vi "Display Lab Panel V5.vi"() -> ()   [LabVIEW 2013]
uses:
  Global display 1.vi
  Global display 2.vi
  Global display 3.vi
panel:
  in  "Tab Control 2":T1(tab)
  out "SIG LAB05-2":T2 {"PF" format="%.2f"; "AMPS" format="%.1f"}
  out "SIG LAB05-1":T2 {"PF" format="%.2f"; "AMPS" format="%.1f"}
  out "SIG LAB04-2":T2 {"PF" format="%.2f"; "AMPS" format="%.1f"}
  out "SIG LAB04-1":T2 {"PF" format="%.2f"; "AMPS" format="%.1f"}
  out "SIG LAB03-2":T2 {"PF" format="%.2f"; "AMPS" format="%.1f"}
  out "SIG LAB03-1":T2 {"PF" format="%.2f"; "AMPS" format="%.1f"}
  out "SIG LAB02-2":T2 {"PF" format="%.2f"; "AMPS" format="%.1f"}
  in  "RUN LAB01-1":bool
  in  "O/I  LAB05-1":bool
  in  "O/I  LAB05-2":bool
  in  "O/I  LAB04-1":bool
  in  "O/I  LAB04-2":bool
  in  "O/I  LAB02-1":bool
  in  "O/I  LAB02-2":bool
  in  "O/I  LAB01-2":bool
  in  "O/I  LAB01-1":bool
  in  "O/I  LAB03-1":bool
  in  "RUN LAB05-2":bool
  in  "RUN LAB05-1":bool
  in  "RUN LAB04-2":bool
  in  "RUN LAB04-1":bool
  in  "RUN LAB03-2":bool
  in  "RUN LAB03-1":bool
  in  "RUN LAB02-2":bool
  in  "RUN LAB02-1":bool
  in  "RUN LAB01-2":bool
  in  "SELECT LAB05-2":T3(radio)
  in  "SELECT LAB05-1":T3(radio)
  in  "SELECT LAB04-2":T3(radio)
  in  "SELECT LAB04-1":T3(radio)
  in  "SELECT LAB03-2":T3(radio)
  in  "SELECT LAB03-1":T3(radio)
  in  "SELECT LAB02-2":T3(radio)
  in  "SELECT LAB02-1":T3(radio)
  in  "SELECT LAB01-2":T3(radio)
  in  "SELECT LAB01-1":T3(radio)
  in  "O/I  LAB03-2":bool
  out "SIG LAB01-1":T2 {"PF" format="%.2f"; "AMPS" format="%.1f"}
  out "SIG LAB01-2":T2 {"PF" format="%.2f"; "AMPS" format="%.1f"}
  out "SIG LAB02-1":T2 {"PF" format="%.2f"; "AMPS" format="%.1f"}
  out "DISP LAB05-2":T4 {"MINS" format="%.2g"}
  out "DISP LAB05-1":T4 {"MINS" format="%.2g"}
  out "DISP LAB04-2":T4 {"MINS" format="%.2g"}
  out "DISP LAB04-1":T4 {"MINS" format="%.2g"}
  out "DISP LAB03-2":T4 {"MINS" format="%.2g"}
  out "DISP LAB03-1":T4 {"MINS" format="%.2g"}
  in  "SET LAB05-2":T5={"NAME"="", "DESCRIPTION"="", "CYCLES"=5.0, "T-RISE mins"=0.0, "T-RISE deg C"=0.0} {"CYCLES" min=5.0 step=1.0}
  in  "SET LAB05-1":T5={"NAME"="", "DESCRIPTION"="", "CYCLES"=5.0, "T-RISE mins"=0.0, "T-RISE deg C"=0.0} {"CYCLES" min=5.0 step=1.0}
  in  "SET LAB04-2":T5={"NAME"="", "DESCRIPTION"="", "CYCLES"=5.0, "T-RISE mins"=0.0, "T-RISE deg C"=0.0} {"CYCLES" min=5.0 step=1.0}
  in  "SET LAB04-1":T5={"NAME"="", "DESCRIPTION"="", "CYCLES"=5.0, "T-RISE mins"=0.0, "T-RISE deg C"=0.0} {"CYCLES" min=5.0 step=1.0}
  in  "SET LAB03-2":T5={"NAME"="", "DESCRIPTION"="", "CYCLES"=5.0, "T-RISE mins"=0.0, "T-RISE deg C"=0.0} {"CYCLES" min=5.0 step=1.0}
  in  "SET LAB03-1":T5={"NAME"="", "DESCRIPTION"="", "CYCLES"=5.0, "T-RISE mins"=0.0, "T-RISE deg C"=0.0} {"CYCLES" min=5.0 step=1.0}
  out "DISP LAB02-2":T4 {"MINS" format="%.2g"}
  out "DISP LAB02-1":T4 {"MINS" format="%.2g"}
  in  "SET LAB02-2":T5={"NAME"="", "DESCRIPTION"="", "CYCLES"=5.0, "T-RISE mins"=0.0, "T-RISE deg C"=0.0} {"CYCLES" min=5.0 step=1.0}
  in  "SET LAB02-1":T5={"NAME"="", "DESCRIPTION"="", "CYCLES"=5.0, "T-RISE mins"=0.0, "T-RISE deg C"=0.0} {"CYCLES" min=5.0 step=1.0}
  out "RESULT LAB05-2":bool
  out "RESULT LAB05-1":bool
  out "RESULT LAB04-2":bool
  out "RESULT LAB04-1":bool
  out "RESULT LAB03-2":bool
  out "RESULT LAB03-1":bool
  out "RESULT LAB02-2":bool
  out "RESULT LAB02-1":bool
  out "RESULT LAB01-2":bool
  out "RESULT LAB01-1":bool
  in  "SET LAB01-1":T5={"NAME"="", "DESCRIPTION"="", "CYCLES"=5.0, "T-RISE mins"=0.0, "T-RISE deg C"=0.0} {"CYCLES" min=5.0 step=1.0}
  in  "SET LAB01-2":T5={"NAME"="", "DESCRIPTION"="", "CYCLES"=5.0, "T-RISE mins"=0.0, "T-RISE deg C"=0.0} {"CYCLES" min=5.0 step=1.0}
  out "DISP LAB01-1":T4 {"MINS" format="%.2g"}
  out "DISP LAB01-2":T4 {"MINS" format="%.2f"}
  in  "Save Log Files\nTo Disk For\nViewing":bool
  out "LOG LAB05-2":string
  out "LOG LAB04-2":string
  out "LOG LAB03-2":string
  out "LOG LAB02-2":string
  out "LOG LAB01-2":string
  out "LOG LAB05-1":string
  out "LOG LAB04-1":string
  out "LOG LAB03-1":string
  out "LOG LAB02-1":string
  out "LOG LAB01-1":string
  out "LAB01 TEMP":dynamicdata(graph)
  out "LAB01 VOLTS":dynamicdata(graph)
  out "LAB01 AMPS":dynamicdata(graph)
  out "LAB02 TEMP":dynamicdata(graph)
  out "LAB02 VOLTS":dynamicdata(graph)
  out "LAB02 AMPS":dynamicdata(graph)
  out "LAB03 TEMP":dynamicdata(graph)
  out "LAB03 VOLTS":dynamicdata(graph)
  out "LAB03 AMPS":dynamicdata(graph)
  out "LAB04 TEMP":dynamicdata(graph)
  out "LAB04 VOLTS":dynamicdata(graph)
  out "LAB04 AMPS":dynamicdata(graph)
  out "LAB05 TEMP":dynamicdata(graph)
  out "LAB05 VOLTS":dynamicdata(graph)
  out "LAB05 AMPS":dynamicdata(graph)
  in  "Stop Button":bool
  out "log file dir":string
  out "log5-2":dbl
  out "log4-2":dbl
  out "log3-2":dbl
  out "log2-2":dbl
  out "log1-2":dbl
  out "log5-1":dbl
  out "log4-1":dbl
  out "log3-1":dbl
  out "log2-1":dbl
  out "log1-1":dbl
  out "graph update":bool
  out "LF5-2":bool
  out "LF5-1":bool
  out "LF3-2":bool
  out "LF3-1":bool
  out "LF4-2":bool
  out "LF4-1":bool
  out "LF2-2":bool
  out "LF2-1":bool
  out "LF1-2":bool
  out "LF1-1":bool
  out "error out":errorcluster
  # "LAB01"
  # "LAB02"
  # "LAB05"
  # "LAB03"
  # "LAB04"
  # "LAB01"
  # "LAB02"
  # "LAB03"
  # "LAB04"
  # "LAB05"
  # "PANEL ID / DATE / TIME / DESCRIPTION / CYCLES / TEST TIME / STATUS"
  # "PANEL ID / DATE / TIME / DESCRIPTION / CYCLES / TEST TIME / STATUS"
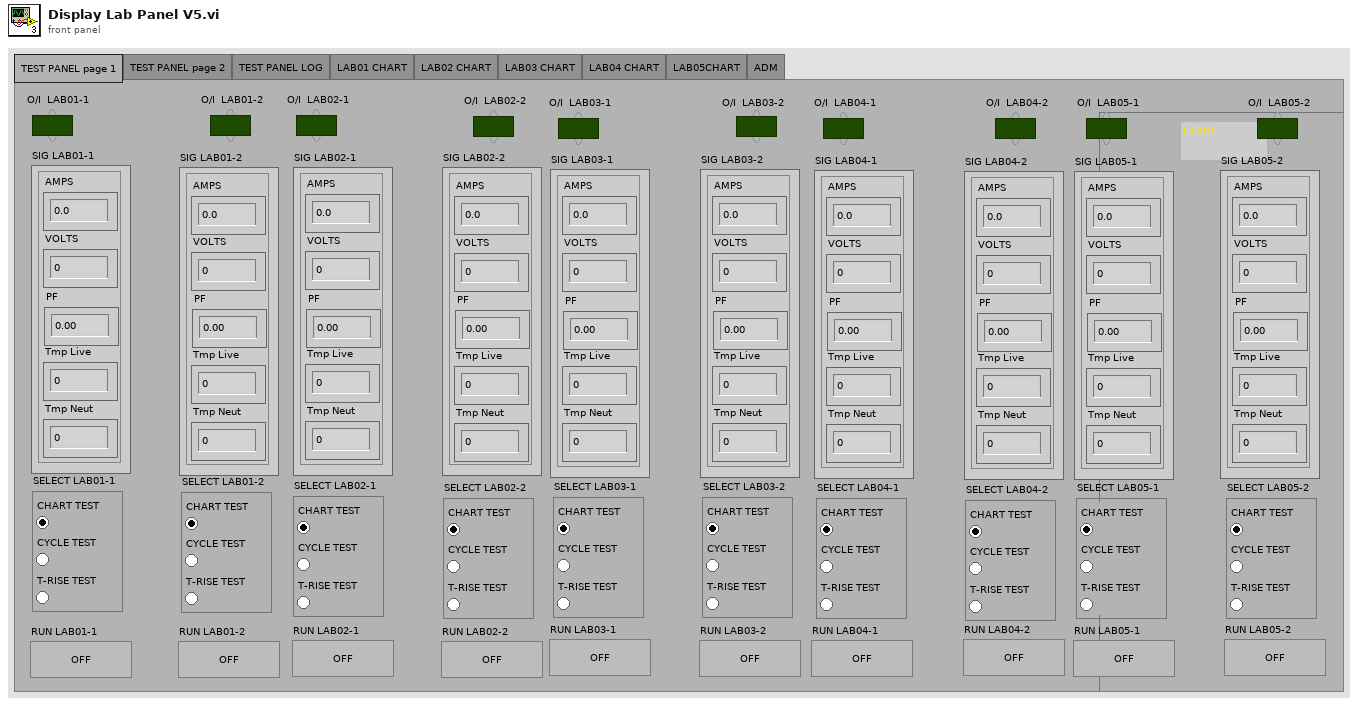
[diagram p1: front panel]
types:
  T1 = enum32{"TEST PANEL page 1", "TEST PANEL page 2", "TEST PANEL LOG", "LAB01 CHART", "LAB02 CHART", "LAB03 CHART", "LAB04 CHART", "LAB05CHART", "ADM"}
  T2 = cluster{"AMPS":dbl, "VOLTS":dbl, "PF":dbl, "Tmp Live":dbl, "Tmp Neut":dbl}
  T3 = enum32{"CHART TEST", "CYCLE TEST", "T-RISE TEST"}
  T4 = cluster{"CYCLE":dbl, "MINS":dbl, "STATUS":string}
  T5 = cluster{"NAME":string, "DESCRIPTION":string, "CYCLES":dbl, "T-RISE mins":dbl, "T-RISE deg C":dbl}
  T6 = enum8{"Enabled", "Disabled", "Disabled and Grayed Out"}
  T7 = cluster{string, "date string":string, "time string":string, "DESCRIPTION":string, string, string, "STATUS":string}
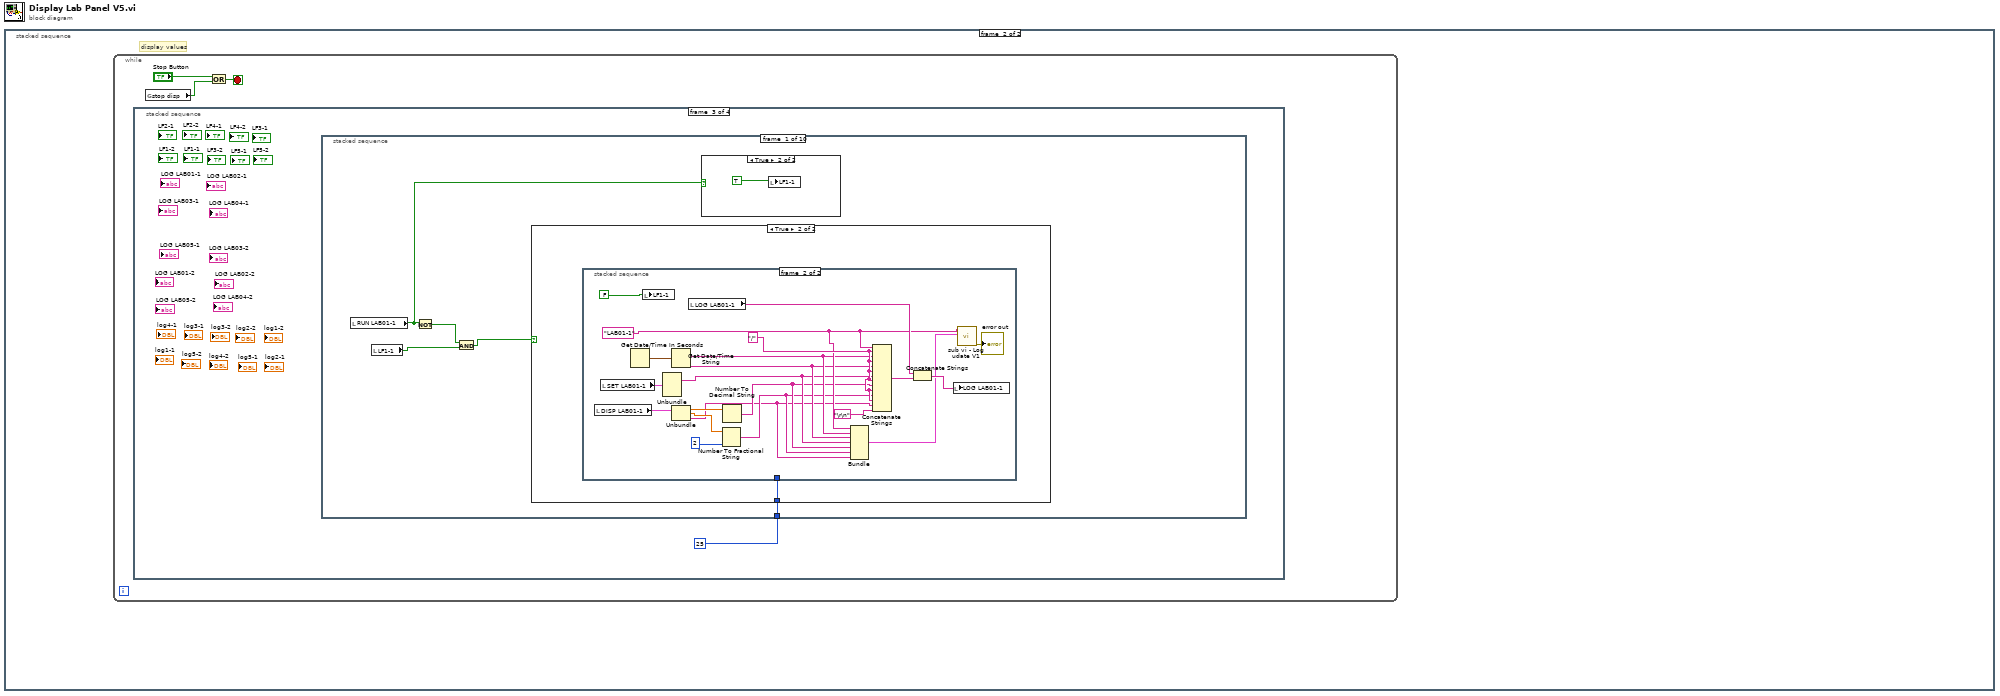
[diagram p0: block diagram]
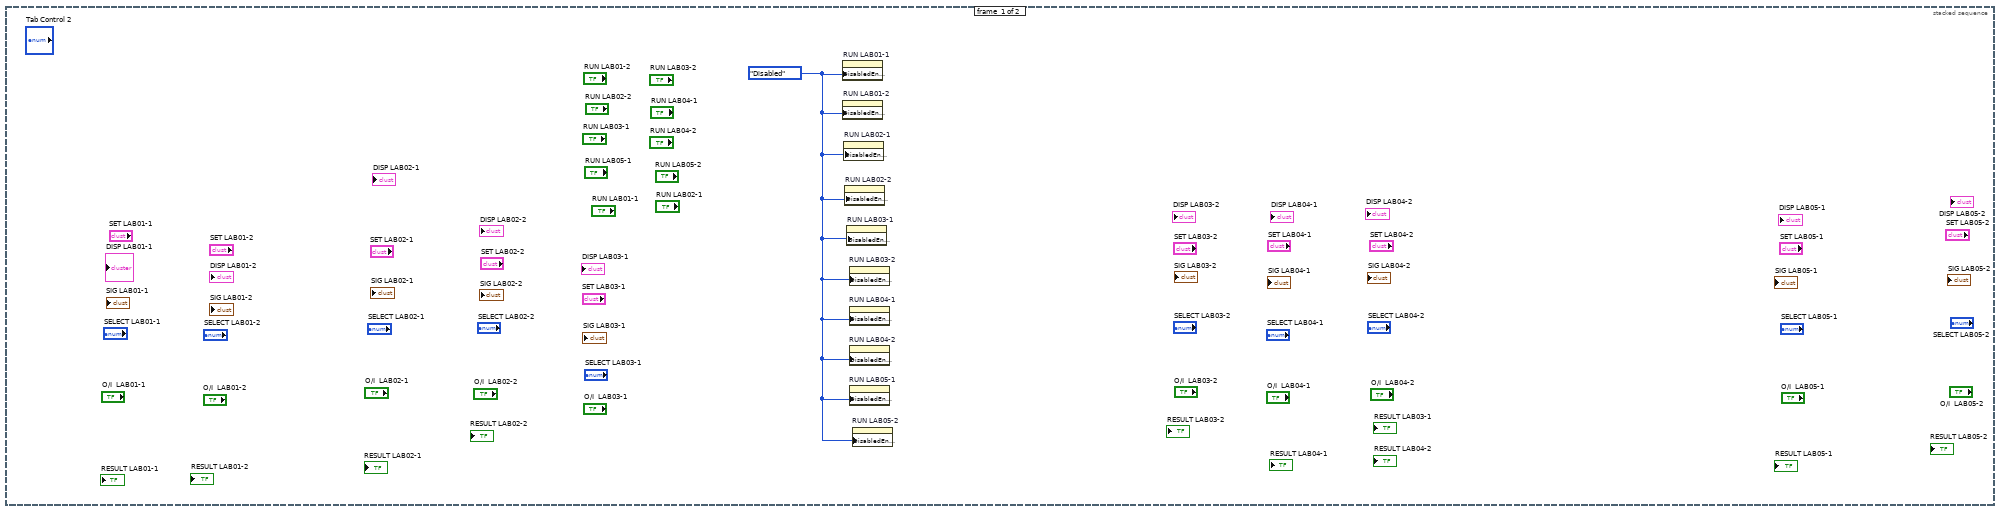
[diagram p2: hidden frame]
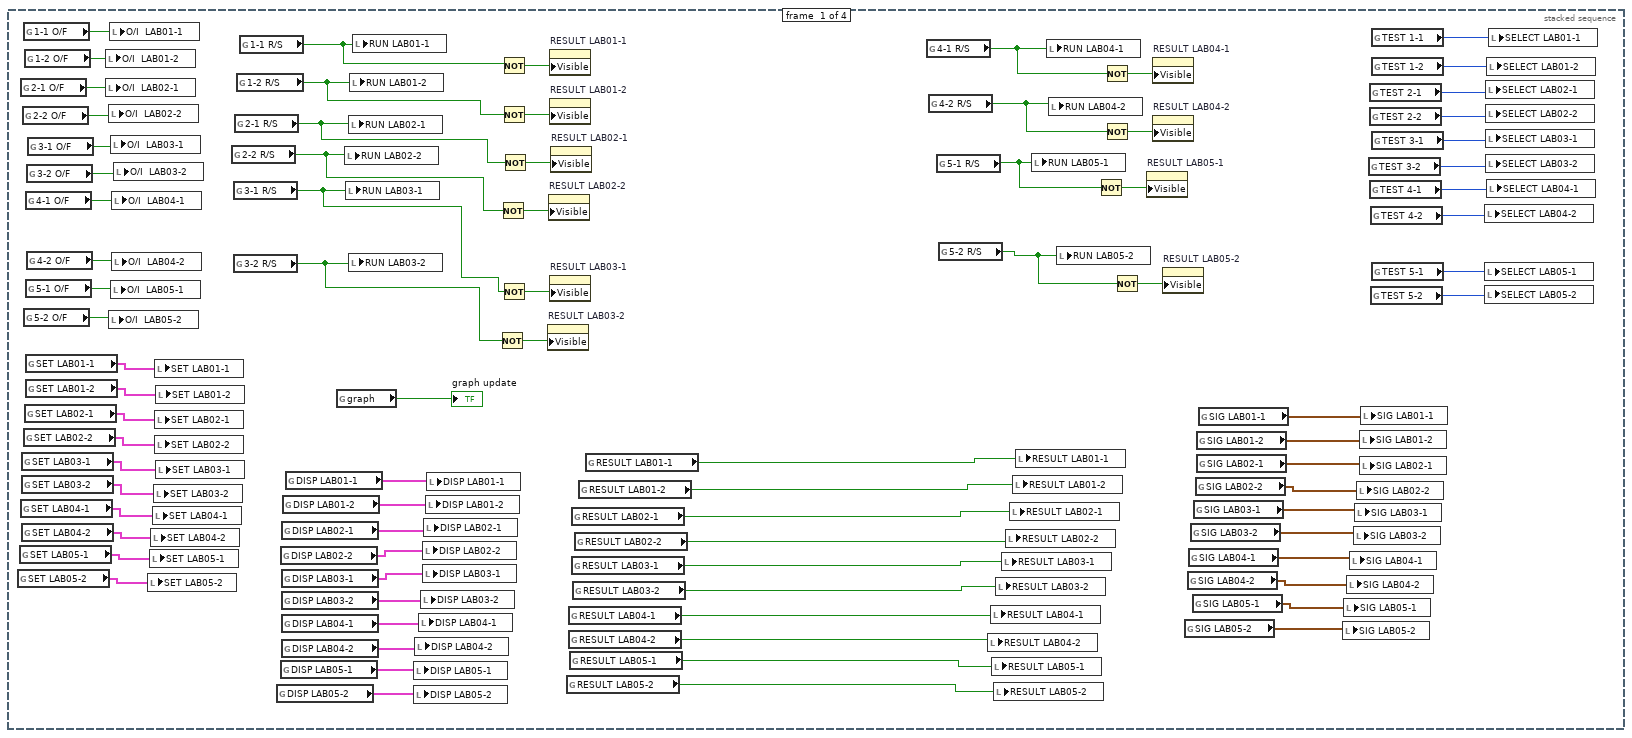
[diagram p3: hidden frame]
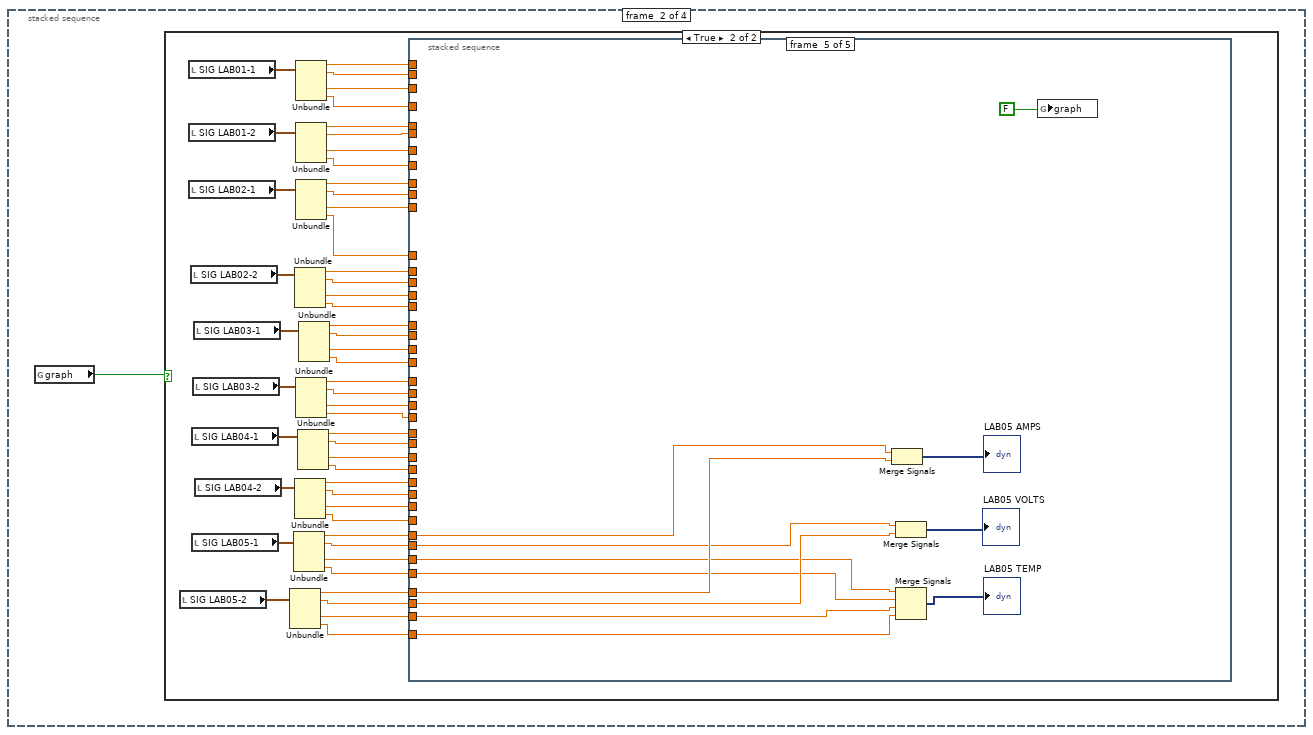
[diagram p4: hidden frame]
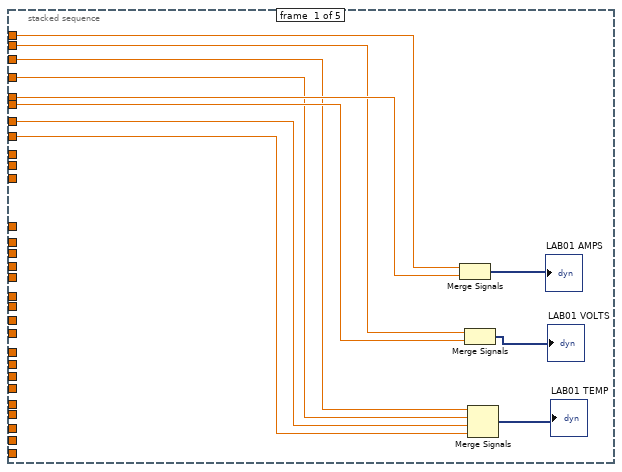
[diagram p6: hidden frame]
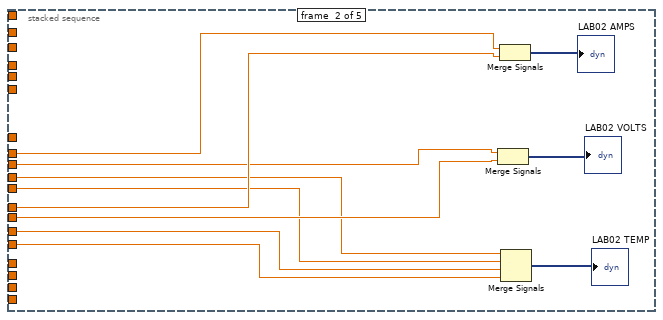
[diagram p7: hidden frame]
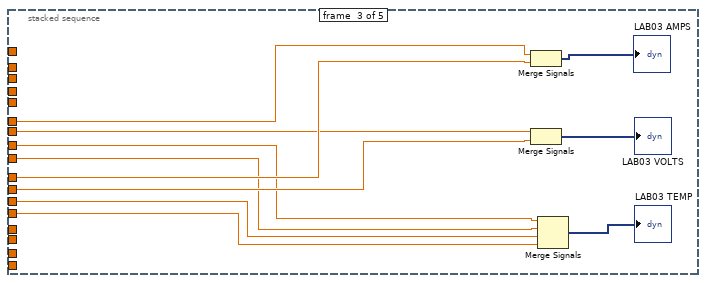
[diagram p8: hidden frame]
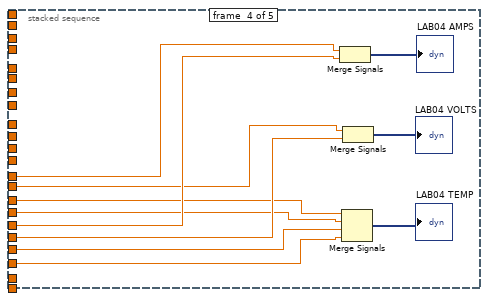
[diagram p9: hidden frame]
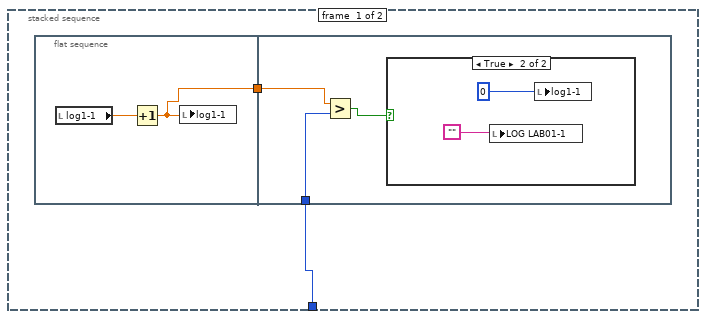
[diagram p11: hidden frame]
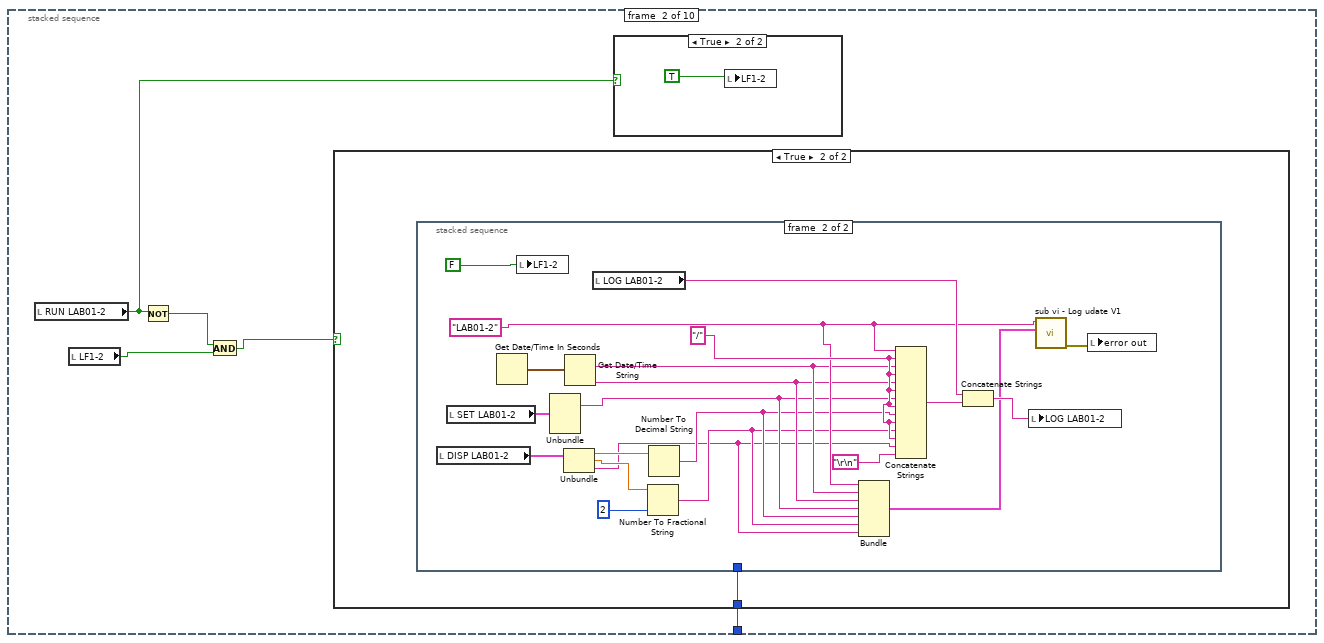
[diagram p14: hidden frame]
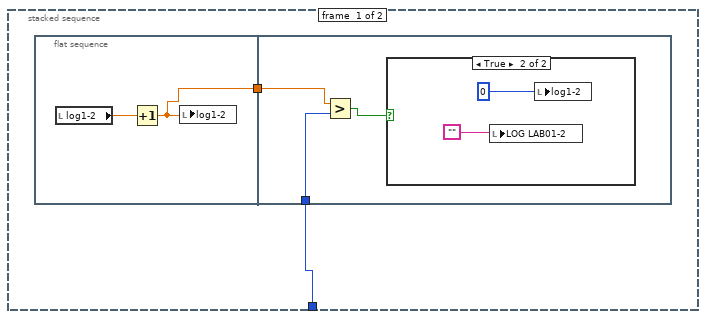
[diagram p16: hidden frame]
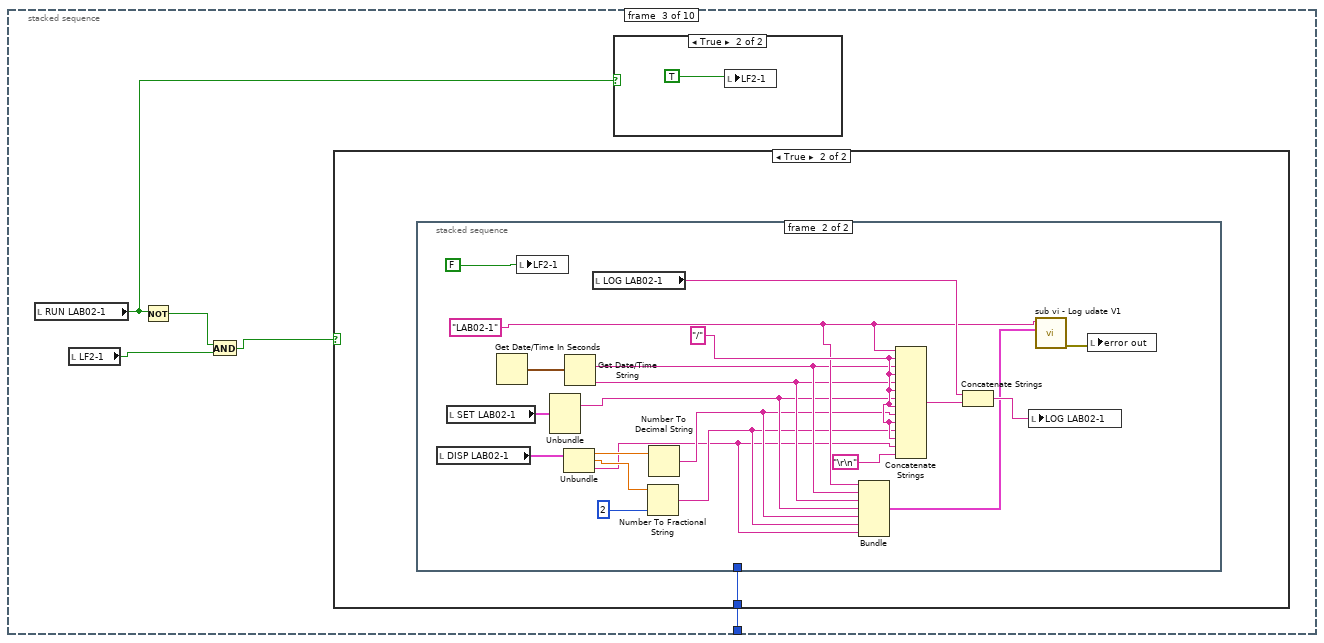
[diagram p19: hidden frame]
diagram:
  n1 = stacked-sequence {
    frame #0 {
      w1 = T6."Disabled" ("Disabled")
      n2 = property on="RUN LAB01-1" class="Bool (strict)"("DisabledEnum"=w1) -> ()  [unwired: 2 in, 2 out]
      n3 = property on="RUN LAB01-2" class="Bool (strict)"("DisabledEnum"=w1) -> ()  [unwired: 2 in, 2 out]
      n4 = property on="RUN LAB02-1" class="Bool (strict)"("DisabledEnum"=w1) -> ()  [unwired: 2 in, 2 out]
      n5 = property on="RUN LAB02-2" class="Bool (strict)"("DisabledEnum"=w1) -> ()  [unwired: 2 in, 2 out]
      n6 = property on="RUN LAB03-1" class="Bool (strict)"("DisabledEnum"=w1) -> ()  [unwired: 2 in, 2 out]
      n7 = property on="RUN LAB03-2" class="Bool (strict)"("DisabledEnum"=w1) -> ()  [unwired: 2 in, 2 out]
      n8 = property on="RUN LAB04-1" class="Bool (strict)"("DisabledEnum"=w1) -> ()  [unwired: 2 in, 2 out]
      n9 = property on="RUN LAB04-2" class="Bool (strict)"("DisabledEnum"=w1) -> ()  [unwired: 2 in, 2 out]
      n10 = property on="RUN LAB05-1" class="Bool (strict)"("DisabledEnum"=w1) -> ()  [unwired: 2 in, 2 out]
      n11 = property on="RUN LAB05-2" class="Bool (strict)"("DisabledEnum"=w1) -> ()  [unwired: 2 in, 2 out]
    }
    frame #1 {
      # "display values"
      n12 = while {
        stop <- w4 stop-if-true
        n13 = stacked-sequence {
          frame #0 {
            n14 = global read "Global display 2.vi" "SET LAB05-2"() -> (w46:T5)
            n15 = global read "Global display 2.vi" "SET LAB05-1"() -> (w47:T5)
            n16 = global read "Global display 1.vi" "2-1 O/F"() -> (w83:bool)
            n17 = global read "Global display 2.vi" "SET LAB04-1"() -> (w49:T5)
            n18 = global read "Global display 2.vi" "SET LAB03-1"() -> (w51:T5)
            n19 = global read "Global display 2.vi" "SET LAB03-2"() -> (w50:T5)
            n20 = global read "Global display 2.vi" "SET LAB04-2"() -> (w48:T5)
            n21 = global read "Global display 1.vi" "2-2 O/F"() -> (w82:bool)
            n22 = global read "Global display 1.vi" "1-1 O/F"() -> (w85:bool)
            n23 = global read "Global display 1.vi" "5-2 O/F"() -> (w76:bool)
            n24 = global read "Global display 2.vi" "SET LAB02-2"() -> (w52:T5)
            n25 = global read "Global display 1.vi" "1-2 O/F"() -> (w84:bool)
            n26 = global read "Global display 2.vi" "SET LAB02-1"() -> (w53:T5)
            n27 = global read "Global display 1.vi" "4-1 O/F"() -> (w79:bool)
            n28 = global read "Global display 1.vi" "5-1 O/F"() -> (w77:bool)
            n29 = global read "Global display 2.vi" "SET LAB01-1"() -> (w55:T5)
            n30 = global read "Global display 2.vi" "SET LAB01-2"() -> (w54:T5)
            n31 = global read "Global display 1.vi" "3-2 O/F"() -> (w80:bool)
            n32 = global read "Global display 1.vi" "4-2 O/F"() -> (w78:bool)
            n33 = global read "Global display 1.vi" "3-1 O/F"() -> (w81:bool)
            n34 = local write "O/I  LAB01-2"(w84) -> ()
            n35 = local write "O/I  LAB02-1"(w83) -> ()
            n36 = local write "O/I  LAB02-2"(w82) -> ()
            n37 = local write "O/I  LAB05-2"(w76) -> ()
            n38 = local write "O/I  LAB01-1"(w85) -> ()
            n39 = local write "O/I  LAB03-1"(w81) -> ()
            n40 = local write "O/I  LAB05-1"(w77) -> ()
            n41 = local write "O/I  LAB04-1"(w79) -> ()
            n42 = local write "O/I  LAB04-2"(w78) -> ()
            n43 = local write "O/I  LAB03-2"(w80) -> ()
            n44 = local write "SET LAB05-2"(w46) -> ()
            n45 = local write "SET LAB05-1"(w47) -> ()
            n46 = local write "SET LAB04-2"(w48) -> ()
            n47 = local write "SET LAB04-1"(w49) -> ()
            n48 = local write "SET LAB03-2"(w50) -> ()
            n49 = local write "SET LAB01-1"(w55) -> ()
            n50 = local write "SET LAB02-1"(w53) -> ()
            n51 = local write "SET LAB02-2"(w52) -> ()
            n52 = local write "SET LAB01-2"(w54) -> ()
            n53 = local write "SET LAB03-1"(w51) -> ()
            n54 = global read "Global display 1.vi" "2-2 R/S"() -> (w16:bool)
            n55 = global read "Global display 1.vi" "3-1 R/S"() -> (w15:bool)
            n56 = global read "Global display 1.vi" "3-2 R/S"() -> (w14:bool)
            n57 = global read "Global display 1.vi" "2-1 R/S"() -> (w17:bool)
            n58 = global read "Global display 1.vi" "1-2 R/S"() -> (w18:bool)
            n59 = global read "Global display 1.vi" "1-1 R/S"() -> (w24:bool)
            n60 = global read "Global display 2.vi" "DISP LAB05-2"() -> (w36:T4)
            n61 = global read "Global display 2.vi" "DISP LAB02-2"() -> (w42:T4)
            n62 = global read "Global display 2.vi" "DISP LAB05-1"() -> (w37:T4)
            n63 = global read "Global display 2.vi" "DISP LAB02-1"() -> (w43:T4)
            n64 = global read "Global display 2.vi" "DISP LAB03-1"() -> (w41:T4)
            n65 = global read "Global display 2.vi" "DISP LAB03-2"() -> (w40:T4)
            n66 = global read "Global display 2.vi" "DISP LAB04-1"() -> (w39:T4)
            n67 = global read "Global display 2.vi" "DISP LAB04-2"() -> (w38:T4)
            n68 = global read "Global display 2.vi" "DISP LAB01-2"() -> (w44:T4)
            n69 = global read "Global display 2.vi" "DISP LAB01-1"() -> (w45:T4)
            n70 = global read "Global display 3.vi" "graph"() -> (→"graph update":bool)
            n71 = local write "RUN LAB02-2"(w16) -> ()
            n72 = local write "RUN LAB03-1"(w15) -> ()
            n73 = local write "RUN LAB02-1"(w17) -> ()
            n74 = local write "RUN LAB03-2"(w14) -> ()
            n75 = local write "RUN LAB01-2"(w18) -> ()
            n76 = local write "RUN LAB01-1"(w24) -> ()
            n77 = local write "DISP LAB05-1"(w37) -> ()
            n78 = local write "DISP LAB05-2"(w36) -> ()
            n79 = local write "DISP LAB04-2"(w38) -> ()
            n80 = local write "DISP LAB04-1"(w39) -> ()
            n81 = local write "DISP LAB03-2"(w40) -> ()
            n82 = local write "DISP LAB02-2"(w42) -> ()
            n83 = local write "DISP LAB03-1"(w41) -> ()
            n84 = local write "DISP LAB02-1"(w43) -> ()
            n85 = local write "DISP LAB01-2"(w44) -> ()
            n86 = local write "DISP LAB01-1"(w45) -> ()
            n87 = Not(x=w14) -> (.not. x?=w19:bool)
            n88 = Not(x=w16) -> (.not. x?=w21:bool)
            n89 = Not(x=w24) -> (.not. x?=w25:bool)
            n90 = Not(x=w18) -> (.not. x?=w23:bool)
            n91 = Not(x=w15) -> (.not. x?=w20:bool)
            n92 = Not(x=w17) -> (.not. x?=w22:bool)
            n93 = property on="RESULT LAB03-2" class="Bool (strict)"("Visible"=w19) -> ()  [unwired: 2 in, 2 out]
            n94 = property on="RESULT LAB02-2" class="Bool (strict)"("Visible"=w21) -> ()  [unwired: 2 in, 2 out]
            n95 = property on="RESULT LAB01-1" class="Bool (strict)"("Visible"=w25) -> ()  [unwired: 2 in, 2 out]
            n96 = property on="RESULT LAB01-2" class="Bool (strict)"("Visible"=w23) -> ()  [unwired: 2 in, 2 out]
            n97 = property on="RESULT LAB03-1" class="Bool (strict)"("Visible"=w20) -> ()  [unwired: 2 in, 2 out]
            n98 = property on="RESULT LAB02-1" class="Bool (strict)"("Visible"=w22) -> ()  [unwired: 2 in, 2 out]
            n99 = global read "Global display 2.vi" "RESULT LAB05-2"() -> (w26:bool)
            n100 = global read "Global display 2.vi" "RESULT LAB04-1"() -> (w29:bool)
            n101 = global read "Global display 2.vi" "RESULT LAB04-2"() -> (w28:bool)
            n102 = global read "Global display 2.vi" "RESULT LAB05-1"() -> (w27:bool)
            n103 = global read "Global display 2.vi" "RESULT LAB02-1"() -> (w33:bool)
            n104 = global read "Global display 2.vi" "RESULT LAB03-1"() -> (w31:bool)
            n105 = global read "Global display 2.vi" "RESULT LAB03-2"() -> (w30:bool)
            n106 = global read "Global display 2.vi" "RESULT LAB02-2"() -> (w32:bool)
            n107 = global read "Global display 2.vi" "RESULT LAB01-2"() -> (w34:bool)
            n108 = global read "Global display 2.vi" "RESULT LAB01-1"() -> (w35:bool)
            n109 = global read "Global display 1.vi" "4-1 R/S"() -> (w12:bool)
            n110 = global read "Global display 1.vi" "4-2 R/S"() -> (w10:bool)
            n111 = global read "Global display 1.vi" "5-1 R/S"() -> (w8:bool)
            n112 = global read "Global display 1.vi" "5-2 R/S"() -> (w6:bool)
            n113 = local write "RESULT LAB04-2"(w28) -> ()
            n114 = local write "RESULT LAB04-1"(w29) -> ()
            n115 = local write "RESULT LAB05-1"(w27) -> ()
            n116 = local write "RESULT LAB05-2"(w26) -> ()
            n117 = local write "RESULT LAB03-2"(w30) -> ()
            n118 = local write "RESULT LAB03-1"(w31) -> ()
            n119 = local write "RESULT LAB02-2"(w32) -> ()
            n120 = local write "RESULT LAB02-1"(w33) -> ()
            n121 = local write "RESULT LAB01-2"(w34) -> ()
            n122 = local write "RESULT LAB01-1"(w35) -> ()
            n123 = local write "RUN LAB05-1"(w8) -> ()
            n124 = local write "RUN LAB04-1"(w12) -> ()
            n125 = local write "RUN LAB04-2"(w10) -> ()
            n126 = local write "RUN LAB05-2"(w6) -> ()
            n127 = Not(x=w8) -> (.not. x?=w9:bool)
            n128 = Not(x=w12) -> (.not. x?=w13:bool)
            n129 = Not(x=w10) -> (.not. x?=w11:bool)
            n130 = Not(x=w6) -> (.not. x?=w7:bool)
            n131 = property on="RESULT LAB05-1" class="Bool (strict)"("Visible"=w9) -> ()  [unwired: 2 in, 2 out]
            n132 = property on="RESULT LAB04-1" class="Bool (strict)"("Visible"=w13) -> ()  [unwired: 2 in, 2 out]
            n133 = property on="RESULT LAB04-2" class="Bool (strict)"("Visible"=w11) -> ()  [unwired: 2 in, 2 out]
            n134 = property on="RESULT LAB05-2" class="Bool (strict)"("Visible"=w7) -> ()  [unwired: 2 in, 2 out]
            n135 = global read "Global display 1.vi" "SIG LAB05-2"() -> (w56:T2)
            n136 = global read "Global display 1.vi" "SIG LAB04-2"() -> (w58:T2)
            n137 = global read "Global display 1.vi" "SIG LAB04-1"() -> (w59:T2)
            n138 = global read "Global display 1.vi" "SIG LAB03-2"() -> (w60:T2)
            n139 = global read "Global display 1.vi" "SIG LAB05-1"() -> (w57:T2)
            n140 = global read "Global display 1.vi" "SIG LAB03-1"() -> (w61:T2)
            n141 = global read "Global display 1.vi" "SIG LAB02-2"() -> (w62:T2)
            n142 = global read "Global display 1.vi" "SIG LAB01-2"() -> (w64:T2)
            n143 = global read "Global display 1.vi" "SIG LAB02-1"() -> (w63:T2)
            n144 = global read "Global display 1.vi" "SIG LAB01-1"() -> (w65:T2)
            n145 = local write "SIG LAB05-2"(w56) -> ()
            n146 = local write "SIG LAB05-1"(w57) -> ()
            n147 = local write "SIG LAB04-2"(w58) -> ()
            n148 = local write "SIG LAB04-1"(w59) -> ()
            n149 = local write "SIG LAB03-2"(w60) -> ()
            n150 = local write "SIG LAB03-1"(w61) -> ()
            n151 = local write "SIG LAB02-2"(w62) -> ()
            n152 = local write "SIG LAB01-2"(w64) -> ()
            n153 = local write "SIG LAB02-1"(w63) -> ()
            n154 = local write "SIG LAB01-1"(w65) -> ()
            n155 = global read "Global display 1.vi" "TEST 3-2"() -> (w70:T3)
            n156 = global read "Global display 1.vi" "TEST 2-1"() -> (w73:T3)
            n157 = global read "Global display 1.vi" "TEST 2-2"() -> (w72:T3)
            n158 = global read "Global display 1.vi" "TEST 4-1"() -> (w69:T3)
            n159 = global read "Global display 1.vi" "TEST 4-2"() -> (w68:T3)
            n160 = global read "Global display 1.vi" "TEST 5-2"() -> (w66:T3)
            n161 = global read "Global display 1.vi" "TEST 1-1"() -> (w75:T3)
            n162 = global read "Global display 1.vi" "TEST 1-2"() -> (w74:T3)
            n163 = global read "Global display 1.vi" "TEST 3-1"() -> (w71:T3)
            n164 = global read "Global display 1.vi" "TEST 5-1"() -> (w67:T3)
            n165 = local write "SELECT LAB04-2"(w68) -> ()
            n166 = local write "SELECT LAB05-1"(w67) -> ()
            n167 = local write "SELECT LAB05-2"(w66) -> ()
            n168 = local write "SELECT LAB02-1"(w73) -> ()
            n169 = local write "SELECT LAB02-2"(w72) -> ()
            n170 = local write "SELECT LAB03-1"(w71) -> ()
            n171 = local write "SELECT LAB03-2"(w70) -> ()
            n172 = local write "SELECT LAB01-2"(w74) -> ()
            n173 = local write "SELECT LAB04-1"(w69) -> ()
            n174 = local write "SELECT LAB01-1"(w75) -> ()
          }
          frame #1 {
            n175 = global read "Global display 3.vi" "graph"() -> (w86:bool)
            n176 = case shown="True" w86 {
              frame False {
              }
              frame True {
                n177 = local read "SIG LAB05-2"() -> (w127:T2)
                n178 = local read "SIG LAB01-1"() -> (w136:T2)
                n179 = local read "SIG LAB01-2"() -> (w135:T2)
                n180 = local read "SIG LAB02-1"() -> (w134:T2)
                n181 = local read "SIG LAB02-2"() -> (w133:T2)
                n182 = local read "SIG LAB04-1"() -> (w130:T2)
                n183 = local read "SIG LAB05-1"() -> (w128:T2)
                n184 = local read "SIG LAB03-2"() -> (w131:T2)
                n185 = local read "SIG LAB03-1"() -> (w132:T2)
                n186 = local read "SIG LAB04-2"() -> (w129:T2)
                n187 = Unbundle(w127) -> ("AMPS"=w117:dbl, "VOLTS"=w107:dbl, "Tmp Live"=w97:dbl, "Tmp Neut"=w87:dbl)  [unwired: 1 out]
                n188 = Unbundle(w128) -> ("AMPS"=w118:dbl, "VOLTS"=w108:dbl, "Tmp Live"=w98:dbl, "Tmp Neut"=w88:dbl)  [unwired: 1 out]
                n189 = Unbundle(w133) -> ("AMPS"=w123:dbl, "VOLTS"=w113:dbl, "Tmp Live"=w103:dbl, "Tmp Neut"=w93:dbl)  [unwired: 1 out]
                n190 = Unbundle(w129) -> ("AMPS"=w119:dbl, "VOLTS"=w109:dbl, "Tmp Live"=w100:dbl, "Tmp Neut"=w89:dbl)  [unwired: 1 out]
                n191 = Unbundle(w136) -> ("AMPS"=w126:dbl, "VOLTS"=w116:dbl, "Tmp Live"=w106:dbl, "Tmp Neut"=w96:dbl)  [unwired: 1 out]
                n192 = Unbundle(w135) -> ("AMPS"=w125:dbl, "VOLTS"=w115:dbl, "Tmp Live"=w105:dbl, "Tmp Neut"=w95:dbl)  [unwired: 1 out]
                n193 = Unbundle(w134) -> ("AMPS"=w124:dbl, "VOLTS"=w114:dbl, "Tmp Live"=w104:dbl, "Tmp Neut"=w94:dbl)  [unwired: 1 out]
                n194 = Unbundle(w131) -> ("AMPS"=w121:dbl, "VOLTS"=w111:dbl, "Tmp Live"=w101:dbl, "Tmp Neut"=w91:dbl)  [unwired: 1 out]
                n195 = Unbundle(w130) -> ("AMPS"=w120:dbl, "VOLTS"=w110:dbl, "Tmp Live"=w99:dbl, "Tmp Neut"=w90:dbl)  [unwired: 1 out]
                n196 = Unbundle(w132) -> ("AMPS"=w122:dbl, "VOLTS"=w112:dbl, "Tmp Live"=w102:dbl, "Tmp Neut"=w92:dbl)  [unwired: 1 out]
                n197 = stacked-sequence {
                  tunnel: w126 -> [w147 _ _ _ _]
                  tunnel: w125 -> [w146 _ _ _ _]
                  tunnel: w124 -> [_ _ _ _ _]
                  tunnel: w123 -> [_ w155 _ _ _]
                  tunnel: w122 -> [_ w154 w166 _ _]
                  tunnel: w121 -> [_ _ w165 _ _]
                  tunnel: w120 -> [_ _ _ w180 _]
                  tunnel: w119 -> [_ _ _ w179 _]
                  tunnel: w118 -> [_ _ _ _ w192]
                  tunnel: w117 -> [_ _ _ _ w191]
                  tunnel: w116 -> [w144 _ _ _ _]
                  tunnel: w115 -> [w143 _ _ _ _]
                  tunnel: w114 -> [_ _ _ _ _]
                  tunnel: w113 -> [_ w153 _ _ _]
                  tunnel: w112 -> [_ w152 w164 _ _]
                  tunnel: w111 -> [_ _ w163 _ _]
                  tunnel: w110 -> [_ _ _ w178 _]
                  tunnel: w109 -> [_ _ _ w177 _]
                  tunnel: w108 -> [_ _ _ _ w190]
                  tunnel: w107 -> [_ _ _ _ w189]
                  tunnel: w106 -> [w140 _ _ _ _]
                  tunnel: w105 -> [w138 _ _ _ _]
                  tunnel: w104 -> [_ _ _ _ _]
                  tunnel: w103 -> [_ w151 _ _ _]
                  tunnel: w102 -> [_ w149 w162 _ _]
                  tunnel: w101 -> [_ _ w160 _ _]
                  tunnel: w100 -> [_ _ _ w174 _]
                  tunnel: w99 -> [_ _ _ w176 _]
                  tunnel: w98 -> [_ _ _ _ w188]
                  tunnel: w97 -> [_ _ _ _ w186]
                  tunnel: w96 -> [w139 _ _ _ _]
                  tunnel: w95 -> [w137 _ _ _ _]
                  tunnel: w94 -> [_ _ _ _ _]
                  tunnel: w93 -> [_ w150 _ _ _]
                  tunnel: w92 -> [_ w148 w161 _ _]
                  tunnel: w91 -> [_ _ w159 _ _]
                  tunnel: w90 -> [_ _ _ w175 _]
                  tunnel: w89 -> [_ _ _ w173 _]
                  tunnel: w88 -> [_ _ _ _ w187]
                  tunnel: w87 -> [_ _ _ _ w185]
                  frame #0 {
                    n198 = Merge Signals(w147, w146) -> (→"LAB01 AMPS":dynamicdata)
                    n199 = Merge Signals(w144, w143) -> (→"LAB01 VOLTS":dynamicdata)
                    n200 = Merge Signals(w140, w139, w138, w137) -> (→"LAB01 TEMP":dynamicdata)
                  }
                  frame #1 {
                    n201 = Merge Signals(w153, w152) -> (→"LAB02 VOLTS":dynamicdata)
                    n202 = Merge Signals(w155, w154) -> (→"LAB02 AMPS":dynamicdata)
                    n203 = Merge Signals(w151, w150, w149, w148) -> (→"LAB02 TEMP":dynamicdata)
                  }
                  frame #2 {
                    n204 = Merge Signals(w166, w165) -> (→"LAB03 AMPS":dynamicdata)
                    n205 = Merge Signals(w164, w163) -> (→"LAB03 VOLTS":dynamicdata)
                    n206 = Merge Signals(w162, w161, w160, w159) -> (→"LAB03 TEMP":dynamicdata)
                  }
                  frame #3 {
                    n207 = Merge Signals(w180, w179) -> (→"LAB04 AMPS":dynamicdata)
                    n208 = Merge Signals(w176, w175, w174, w173) -> (→"LAB04 TEMP":dynamicdata)
                    n209 = Merge Signals(w178, w177) -> (→"LAB04 VOLTS":dynamicdata)
                  }
                  frame #4 {
                    n210 = Merge Signals(w192, w191) -> (→"LAB05 AMPS":dynamicdata)
                    n211 = Merge Signals(w190, w189) -> (→"LAB05 VOLTS":dynamicdata)
                    n212 = Merge Signals(w188, w187, w186, w185) -> (→"LAB05 TEMP":dynamicdata)
                    n213 = global write "Global display 3.vi" "graph"(FALSE) -> ()
                  }
                }
              }
            }
          }
          frame #2 {
            n214 = stacked-sequence {
              tunnel: 25 -> [w194 w231 w268 w305 w342 w379 w416 w453 w490 w527]
              frame #0 {
                n215 = local read "RUN LAB01-1"() -> (w195:bool)
                n216 = local read "LF1-1"() -> (w197:bool)
                n217 = Not(x=w195) -> (.not. x?=w198:bool)
                n218 = And(x=w198, y=w197) -> (x .and. y?=w196:bool)
                n219 = case shown="True" w196 {
                  tunnel: w194 -> [_ w199]
                  frame False {
                  }
                  frame True {
                    n220 = stacked-sequence {
                      tunnel: w199 -> [w200 _]
                      frame #0 {
                        n221 = flat-sequence {
                          tunnel: [w202] -> w201
                          tunnel: w201 -> [w205]
                          tunnel: w200 -> [w204]
                          frame #0 {
                            n222 = local read "log1-1"() -> (w203:dbl)
                            n223 = Increment(x=w203) -> (x+1=w202:dbl)
                            n224 = local write "log1-1"(w202) -> ()
                          }
                          frame #1 {
                            n225 = Greater?(x=w205, y=w204) -> (0:w206:bool)
                            n226 = case shown="True" w206 {
                              frame False {
                              }
                              frame True {
                                n227 = local write "LOG LAB01-1"("") -> ()
                                n228 = local write "log1-1"(0) -> ()
                              }
                            }
                          }
                        }
                      }
                      frame #1 {
                        w217 = "LAB01-1"
                        w221 = "/"
                        n229 = local read "DISP LAB01-1"() -> (w228:T4)
                        n230 = local read "SET LAB01-1"() -> (w222:T5)
                        n231 = Get Date/Time In Seconds() -> (seconds since 1Jan1904=w224:timestamp)
                        n232 = local write "LF1-1"(FALSE) -> ()
                        n233 = Unbundle(w222) -> ("DESCRIPTION"=w214:string)  [unwired: 4 out]
                        n234 = Unbundle(w228) -> ("CYCLE"=w227:dbl, "MINS"=w226:dbl, "STATUS"=w211:string)
                        n235 = Get Date/Time String(seconds (now)=w224) -> (date string=w216:string, time string=w215:string)  [unwired: 2 in]
                        n236 = local read "LOG LAB01-1"() -> (w220:string)
                        n237 = Number To Fractional String(number=w226, precision (6)=2) -> (F-format string=w212:string)  [unwired: 2 in]
                        n238 = Number To Decimal String(number=w227) -> (decimal integer string=w213:string)  [unwired: 1 in]
                        n239 = Bundle(w217, "date string"=w216, "time string"=w215, "DESCRIPTION"=w214, w213, w212, "STATUS"=w211) -> (w210:T7)  [unwired: 1 in]
                        n240 = Concatenate Strings(w217, w221, w216, w221, w215, w221, w214, w221, w213, w221, w212, w221, w211, "\r\n") -> (w218:string)
                        n241 = Concatenate Strings(w220, w218) -> (w219:string)
                        n242 = local write "LOG LAB01-1"(w219) -> ()
                        n243 = call "sub vi - Log udate V1.vi"("data"=w210, "panel id"=w217) -> ("error out"=→"error out":errorcluster)  [unwired: 9 in]
                      }
                    }
                  }
                }
                n244 = case shown="True" w195 {
                  frame False {
                  }
                  frame True {
                    n245 = local write "LF1-1"(TRUE) -> ()
                  }
                }
              }
              frame #1 {
                n246 = local read "RUN LAB01-2"() -> (w232:bool)
                n247 = local read "LF1-2"() -> (w234:bool)
                n248 = Not(x=w232) -> (.not. x?=w235:bool)
                n249 = And(x=w235, y=w234) -> (x .and. y?=w233:bool)
                n250 = case shown="True" w233 {
                  tunnel: w231 -> [_ w236]
                  frame False {
                  }
                  frame True {
                    n251 = stacked-sequence {
                      tunnel: w236 -> [w237 _]
                      frame #0 {
                        n252 = flat-sequence {
                          tunnel: [w239] -> w238
                          tunnel: w238 -> [w242]
                          tunnel: w237 -> [w241]
                          frame #0 {
                            n253 = local read "log1-2"() -> (w240:dbl)
                            n254 = Increment(x=w240) -> (x+1=w239:dbl)
                            n255 = local write "log1-2"(w239) -> ()
                          }
                          frame #1 {
                            n256 = Greater?(x=w242, y=w241) -> (0:w243:bool)
                            n257 = case shown="True" w243 {
                              frame False {
                              }
                              frame True {
                                n258 = local write "LOG LAB01-2"("") -> ()
                                n259 = local write "log1-2"(0) -> ()
                              }
                            }
                          }
                        }
                      }
                      frame #1 {
                        w254 = "LAB01-2"
                        w258 = "/"
                        n260 = local read "DISP LAB01-2"() -> (w265:T4)
                        n261 = local read "SET LAB01-2"() -> (w259:T5)
                        n262 = Get Date/Time In Seconds() -> (seconds since 1Jan1904=w261:timestamp)
                        n263 = local write "LF1-2"(FALSE) -> ()
                        n264 = Unbundle(w259) -> ("DESCRIPTION"=w251:string)  [unwired: 4 out]
                        n265 = Unbundle(w265) -> ("CYCLE"=w264:dbl, "MINS"=w263:dbl, "STATUS"=w248:string)
                        n266 = Get Date/Time String(seconds (now)=w261) -> (date string=w253:string, time string=w252:string)  [unwired: 2 in]
                        n267 = local read "LOG LAB01-2"() -> (w257:string)
                        n268 = Number To Fractional String(number=w263, precision (6)=2) -> (F-format string=w249:string)  [unwired: 2 in]
                        n269 = Number To Decimal String(number=w264) -> (decimal integer string=w250:string)  [unwired: 1 in]
                        n270 = Bundle(w254, "date string"=w253, "time string"=w252, "DESCRIPTION"=w251, w250, w249, "STATUS"=w248) -> (w247:T7)  [unwired: 1 in]
                        n271 = Concatenate Strings(w254, w258, w253, w258, w252, w258, w251, w258, w250, w258, w249, w258, w248, "\r\n") -> (w255:string)
                        n272 = Concatenate Strings(w257, w255) -> (w256:string)
                        n273 = local write "LOG LAB01-2"(w256) -> ()
                        n274 = call "sub vi - Log udate V1.vi"("data"=w247, "panel id"=w254) -> ("error out"=w246:errorcluster)  [unwired: 9 in]
                        n275 = local write "error out"(w246) -> ()
                      }
                    }
                  }
                }
                n276 = case shown="True" w232 {
                  frame False {
                  }
                  frame True {
                    n277 = local write "LF1-2"(TRUE) -> ()
                  }
                }
              }
              frame #2 {
                n278 = local read "RUN LAB02-1"() -> (w269:bool)
                n279 = local read "LF2-1"() -> (w271:bool)
                n280 = Not(x=w269) -> (.not. x?=w272:bool)
                n281 = And(x=w272, y=w271) -> (x .and. y?=w270:bool)
                n282 = case shown="True" w270 {
                  tunnel: w268 -> [_ w273]
                  frame False {
                  }
                  frame True {
                    n283 = stacked-sequence {
                      tunnel: w273 -> [w274 _]
                      frame #0 {
                        n284 = flat-sequence {
                          tunnel: [w276] -> w275
                          tunnel: w275 -> [w279]
                          tunnel: w274 -> [w278]
                          frame #0 {
                            n285 = local read "log2-1"() -> (w277:dbl)
                            n286 = Increment(x=w277) -> (x+1=w276:dbl)
                            n287 = local write "log2-1"(w276) -> ()
                          }
                          frame #1 {
                            n288 = Greater?(x=w279, y=w278) -> (0:w280:bool)
                            n289 = case shown="True" w280 {
                              frame False {
                              }
                              frame True {
                                n290 = local write "LOG LAB02-1"("") -> ()
                                n291 = local write "log2-1"(0) -> ()
                              }
                            }
                          }
                        }
                      }
                      frame #1 {
                        w291 = "LAB02-1"
                        w295 = "/"
                        n292 = local read "DISP LAB02-1"() -> (w302:T4)
                        n293 = local read "SET LAB02-1"() -> (w296:T5)
                        n294 = Get Date/Time In Seconds() -> (seconds since 1Jan1904=w298:timestamp)
                        n295 = local write "LF2-1"(FALSE) -> ()
                        n296 = Unbundle(w296) -> ("DESCRIPTION"=w288:string)  [unwired: 4 out]
                        n297 = Unbundle(w302) -> ("CYCLE"=w301:dbl, "MINS"=w300:dbl, "STATUS"=w285:string)
                        n298 = Get Date/Time String(seconds (now)=w298) -> (date string=w290:string, time string=w289:string)  [unwired: 2 in]
                        n299 = local read "LOG LAB02-1"() -> (w294:string)
                        n300 = Number To Fractional String(number=w300, precision (6)=2) -> (F-format string=w286:string)  [unwired: 2 in]
                        n301 = Number To Decimal String(number=w301) -> (decimal integer string=w287:string)  [unwired: 1 in]
                        n302 = Bundle(w291, "date string"=w290, "time string"=w289, "DESCRIPTION"=w288, w287, w286, "STATUS"=w285) -> (w284:T7)  [unwired: 1 in]
                        n303 = Concatenate Strings(w291, w295, w290, w295, w289, w295, w288, w295, w287, w295, w286, w295, w285, "\r\n") -> (w292:string)
                        n304 = Concatenate Strings(w294, w292) -> (w293:string)
                        n305 = local write "LOG LAB02-1"(w293) -> ()
                        n306 = call "sub vi - Log udate V1.vi"("data"=w284, "panel id"=w291) -> ("error out"=w283:errorcluster)  [unwired: 9 in]
                        n307 = local write "error out"(w283) -> ()
                      }
                    }
                  }
                }
                n308 = case shown="True" w269 {
                  frame False {
                  }
                  frame True {
                    n309 = local write "LF2-1"(TRUE) -> ()
                  }
                }
              }
              frame #3 {
                n310 = local read "RUN LAB02-2"() -> (w306:bool)
                n311 = local read "LF2-2"() -> (w308:bool)
                n312 = Not(x=w306) -> (.not. x?=w309:bool)
                n313 = And(x=w309, y=w308) -> (x .and. y?=w307:bool)
                n314 = case shown="True" w307 {
                  tunnel: w305 -> [_ w310]
                  frame False {
                  }
                  frame True {
                    n315 = stacked-sequence {
                      tunnel: w310 -> [w311 _]
                      frame #0 {
                        n316 = flat-sequence {
                          tunnel: [w313] -> w312
                          tunnel: w312 -> [w316]
                          tunnel: w311 -> [w315]
                          frame #0 {
                            n317 = local read "log2-2"() -> (w314:dbl)
                            n318 = Increment(x=w314) -> (x+1=w313:dbl)
                            n319 = local write "log2-2"(w313) -> ()
                          }
                          frame #1 {
                            n320 = Greater?(x=w316, y=w315) -> (0:w317:bool)
                            n321 = case shown="True" w317 {
                              frame False {
                              }
                              frame True {
                                n322 = local write "LOG LAB02-2"("") -> ()
                                n323 = local write "log2-2"(0) -> ()
                              }
                            }
                          }
                        }
                      }
                      frame #1 {
                        w328 = "LAB02-2"
                        w332 = "/"
                        n324 = local read "DISP LAB02-2"() -> (w339:T4)
                        n325 = local read "SET LAB02-2"() -> (w333:T5)
                        n326 = Get Date/Time In Seconds() -> (seconds since 1Jan1904=w335:timestamp)
                        n327 = local write "LF2-2"(FALSE) -> ()
                        n328 = Unbundle(w333) -> ("DESCRIPTION"=w325:string)  [unwired: 4 out]
                        n329 = Unbundle(w339) -> ("CYCLE"=w338:dbl, "MINS"=w337:dbl, "STATUS"=w322:string)
                        n330 = Get Date/Time String(seconds (now)=w335) -> (date string=w327:string, time string=w326:string)  [unwired: 2 in]
                        n331 = local read "LOG LAB02-2"() -> (w331:string)
                        n332 = Number To Fractional String(number=w337, precision (6)=2) -> (F-format string=w323:string)  [unwired: 2 in]
                        n333 = Number To Decimal String(number=w338) -> (decimal integer string=w324:string)  [unwired: 1 in]
                        n334 = Bundle(w328, "date string"=w327, "time string"=w326, "DESCRIPTION"=w325, w324, w323, "STATUS"=w322) -> (w321:T7)  [unwired: 1 in]
                        n335 = Concatenate Strings(w328, w332, w327, w332, w326, w332, w325, w332, w324, w332, w323, w332, w322, "\r\n") -> (w329:string)
                        n336 = Concatenate Strings(w331, w329) -> (w330:string)
                        n337 = local write "LOG LAB02-2"(w330) -> ()
                        n338 = call "sub vi - Log udate V1.vi"("data"=w321, "panel id"=w328) -> ("error out"=w320:errorcluster)  [unwired: 9 in]
                        n339 = local write "error out"(w320) -> ()
                      }
                    }
                  }
                }
                n340 = case shown="True" w306 {
                  frame False {
                  }
                  frame True {
                    n341 = local write "LF2-2"(TRUE) -> ()
                  }
                }
              }
              frame #4 {
                n342 = local read "RUN LAB03-1"() -> (w343:bool)
                n343 = local read "LF3-1"() -> (w345:bool)
                n344 = Not(x=w343) -> (.not. x?=w346:bool)
                n345 = And(x=w346, y=w345) -> (x .and. y?=w344:bool)
                n346 = case shown="True" w344 {
                  tunnel: w342 -> [_ w347]
                  frame False {
                  }
                  frame True {
                    n347 = stacked-sequence {
                      tunnel: w347 -> [w348 _]
                      frame #0 {
                        n348 = flat-sequence {
                          tunnel: [w350] -> w349
                          tunnel: w349 -> [w353]
                          tunnel: w348 -> [w352]
                          frame #0 {
                            n349 = local read "log3-1"() -> (w351:dbl)
                            n350 = Increment(x=w351) -> (x+1=w350:dbl)
                            n351 = local write "log3-1"(w350) -> ()
                          }
                          frame #1 {
                            n352 = Greater?(x=w353, y=w352) -> (0:w354:bool)
                            n353 = case shown="True" w354 {
                              frame False {
                              }
                              frame True {
                                n354 = local write "LOG LAB03-1"("") -> ()
                                n355 = local write "log3-1"(0) -> ()
                              }
                            }
                          }
                        }
                      }
                      frame #1 {
                        w365 = "LAB03-1"
                        w369 = "/"
                        n356 = local read "DISP LAB03-1"() -> (w376:T4)
                        n357 = local read "SET LAB03-1"() -> (w370:T5)
                        n358 = Get Date/Time In Seconds() -> (seconds since 1Jan1904=w372:timestamp)
                        n359 = local write "LF3-1"(FALSE) -> ()
                        n360 = Unbundle(w370) -> ("DESCRIPTION"=w362:string)  [unwired: 4 out]
                        n361 = Unbundle(w376) -> ("CYCLE"=w375:dbl, "MINS"=w374:dbl, "STATUS"=w359:string)
                        n362 = Get Date/Time String(seconds (now)=w372) -> (date string=w364:string, time string=w363:string)  [unwired: 2 in]
                        n363 = local read "LOG LAB03-1"() -> (w368:string)
                        n364 = Number To Fractional String(number=w374, precision (6)=2) -> (F-format string=w360:string)  [unwired: 2 in]
                        n365 = Number To Decimal String(number=w375) -> (decimal integer string=w361:string)  [unwired: 1 in]
                        n366 = Bundle(w365, "date string"=w364, "time string"=w363, "DESCRIPTION"=w362, w361, w360, "STATUS"=w359) -> (w358:T7)  [unwired: 1 in]
                        n367 = Concatenate Strings(w365, w369, w364, w369, w363, w369, w362, w369, w361, w369, w360, w369, w359, "\r\n") -> (w366:string)
                        n368 = Concatenate Strings(w368, w366) -> (w367:string)
                        n369 = local write "LOG LAB03-1"(w367) -> ()
                        n370 = call "sub vi - Log udate V1.vi"("data"=w358, "panel id"=w365) -> ("error out"=w357:errorcluster)  [unwired: 9 in]
                        n371 = local write "error out"(w357) -> ()
                      }
                    }
                  }
                }
                n372 = case shown="True" w343 {
                  frame False {
                  }
                  frame True {
                    n373 = local write "LF3-1"(TRUE) -> ()
                  }
                }
              }
              frame #5 {
                n374 = local read "RUN LAB03-2"() -> (w380:bool)
                n375 = local read "LF3-2"() -> (w382:bool)
                n376 = Not(x=w380) -> (.not. x?=w383:bool)
                n377 = And(x=w383, y=w382) -> (x .and. y?=w381:bool)
                n378 = case shown="True" w381 {
                  tunnel: w379 -> [_ w384]
                  frame False {
                  }
                  frame True {
                    n379 = stacked-sequence {
                      tunnel: w384 -> [w385 _]
                      frame #0 {
                        n380 = flat-sequence {
                          tunnel: [w387] -> w386
                          tunnel: w386 -> [w390]
                          tunnel: w385 -> [w389]
                          frame #0 {
                            n381 = local read "log3-2"() -> (w388:dbl)
                            n382 = Increment(x=w388) -> (x+1=w387:dbl)
                            n383 = local write "log3-2"(w387) -> ()
                          }
                          frame #1 {
                            n384 = Greater?(x=w390, y=w389) -> (0:w391:bool)
                            n385 = case shown="True" w391 {
                              frame False {
                              }
                              frame True {
                                n386 = local write "LOG LAB03-2"("") -> ()
                                n387 = local write "log3-2"(0) -> ()
                              }
                            }
                          }
                        }
                      }
                      frame #1 {
                        w402 = "LAB03-2"
                        w406 = "/"
                        n388 = local read "DISP LAB03-2"() -> (w413:T4)
                        n389 = local read "SET LAB03-2"() -> (w407:T5)
                        n390 = Get Date/Time In Seconds() -> (seconds since 1Jan1904=w409:timestamp)
                        n391 = local write "LF3-2"(FALSE) -> ()
                        n392 = Unbundle(w407) -> ("DESCRIPTION"=w399:string)  [unwired: 4 out]
                        n393 = Unbundle(w413) -> ("CYCLE"=w412:dbl, "MINS"=w411:dbl, "STATUS"=w396:string)
                        n394 = Get Date/Time String(seconds (now)=w409) -> (date string=w401:string, time string=w400:string)  [unwired: 2 in]
                        n395 = local read "LOG LAB03-2"() -> (w405:string)
                        n396 = Number To Fractional String(number=w411, precision (6)=2) -> (F-format string=w397:string)  [unwired: 2 in]
                        n397 = Number To Decimal String(number=w412) -> (decimal integer string=w398:string)  [unwired: 1 in]
                        n398 = Bundle(w402, "date string"=w401, "time string"=w400, "DESCRIPTION"=w399, w398, w397, "STATUS"=w396) -> (w395:T7)  [unwired: 1 in]
                        n399 = Concatenate Strings(w402, w406, w401, w406, w400, w406, w399, w406, w398, w406, w397, w406, w396, "\r\n") -> (w403:string)
                        n400 = Concatenate Strings(w405, w403) -> (w404:string)
                        n401 = local write "LOG LAB03-2"(w404) -> ()
                        n402 = call "sub vi - Log udate V1.vi"("data"=w395, "panel id"=w402) -> ("error out"=w394:errorcluster)  [unwired: 9 in]
                        n403 = local write "error out"(w394) -> ()
                      }
                    }
                  }
                }
                n404 = case shown="True" w380 {
                  frame False {
                  }
                  frame True {
                    n405 = local write "LF3-2"(TRUE) -> ()
                  }
                }
              }
              frame #6 {
                n406 = local read "RUN LAB04-1"() -> (w417:bool)
                n407 = local read "LF4-1"() -> (w419:bool)
                n408 = Not(x=w417) -> (.not. x?=w420:bool)
                n409 = And(x=w420, y=w419) -> (x .and. y?=w418:bool)
                n410 = case shown="True" w418 {
                  tunnel: w416 -> [_ w421]
                  frame False {
                  }
                  frame True {
                    n411 = stacked-sequence {
                      tunnel: w421 -> [w422 _]
                      frame #0 {
                        n412 = flat-sequence {
                          tunnel: [w424] -> w423
                          tunnel: w423 -> [w427]
                          tunnel: w422 -> [w426]
                          frame #0 {
                            n413 = local read "log4-1"() -> (w425:dbl)
                            n414 = Increment(x=w425) -> (x+1=w424:dbl)
                            n415 = local write "log4-1"(w424) -> ()
                          }
                          frame #1 {
                            n416 = Greater?(x=w427, y=w426) -> (0:w428:bool)
                            n417 = case shown="True" w428 {
                              frame False {
                              }
                              frame True {
                                n418 = local write "LOG LAB04-1"("") -> ()
                                n419 = local write "log4-1"(0) -> ()
                              }
                            }
                          }
                        }
                      }
                      frame #1 {
                        w439 = "LAB04-1"
                        w443 = "/"
                        n420 = local read "DISP LAB04-1"() -> (w450:T4)
                        n421 = local read "SET LAB04-1"() -> (w444:T5)
                        n422 = Get Date/Time In Seconds() -> (seconds since 1Jan1904=w446:timestamp)
                        n423 = local write "LF4-1"(FALSE) -> ()
                        n424 = Unbundle(w444) -> ("DESCRIPTION"=w436:string)  [unwired: 4 out]
                        n425 = Unbundle(w450) -> ("CYCLE"=w449:dbl, "MINS"=w448:dbl, "STATUS"=w433:string)
                        n426 = Get Date/Time String(seconds (now)=w446) -> (date string=w438:string, time string=w437:string)  [unwired: 2 in]
                        n427 = local read "LOG LAB04-1"() -> (w442:string)
                        n428 = Number To Fractional String(number=w448, precision (6)=2) -> (F-format string=w434:string)  [unwired: 2 in]
                        n429 = Number To Decimal String(number=w449) -> (decimal integer string=w435:string)  [unwired: 1 in]
                        n430 = Bundle(w439, "date string"=w438, "time string"=w437, "DESCRIPTION"=w436, w435, w434, "STATUS"=w433) -> (w432:T7)  [unwired: 1 in]
                        n431 = Concatenate Strings(w439, w443, w438, w443, w437, w443, w436, w443, w435, w443, w434, w443, w433, "\r\n") -> (w440:string)
                        n432 = Concatenate Strings(w442, w440) -> (w441:string)
                        n433 = local write "LOG LAB04-1"(w441) -> ()
                        n434 = call "sub vi - Log udate V1.vi"("data"=w432, "panel id"=w439) -> ("error out"=w431:errorcluster)  [unwired: 9 in]
                        n435 = local write "error out"(w431) -> ()
                      }
                    }
                  }
                }
                n436 = case shown="True" w417 {
                  frame False {
                  }
                  frame True {
                    n437 = local write "LF4-1"(TRUE) -> ()
                  }
                }
              }
              frame #7 {
                n438 = local read "RUN LAB04-2"() -> (w454:bool)
                n439 = local read "LF4-2"() -> (w456:bool)
                n440 = Not(x=w454) -> (.not. x?=w457:bool)
                n441 = And(x=w457, y=w456) -> (x .and. y?=w455:bool)
                n442 = case shown="True" w455 {
                  tunnel: w453 -> [_ w458]
                  frame False {
                  }
                  frame True {
                    n443 = stacked-sequence {
                      tunnel: w458 -> [w459 _]
                      frame #0 {
                        n444 = flat-sequence {
                          tunnel: [w461] -> w460
                          tunnel: w460 -> [w464]
                          tunnel: w459 -> [w463]
                          frame #0 {
                            n445 = local read "log4-2"() -> (w462:dbl)
                            n446 = Increment(x=w462) -> (x+1=w461:dbl)
                            n447 = local write "log4-2"(w461) -> ()
                          }
                          frame #1 {
                            n448 = Greater?(x=w464, y=w463) -> (0:w465:bool)
                            n449 = case shown="True" w465 {
                              frame False {
                              }
                              frame True {
                                n450 = local write "LOG LAB04-2"("") -> ()
                                n451 = local write "log4-2"(0) -> ()
                              }
                            }
                          }
                        }
                      }
                      frame #1 {
                        w476 = "LAB04-2"
                        w480 = "/"
                        n452 = local read "DISP LAB04-2"() -> (w487:T4)
                        n453 = local read "SET LAB04-2"() -> (w481:T5)
                        n454 = Get Date/Time In Seconds() -> (seconds since 1Jan1904=w483:timestamp)
                        n455 = local write "LF4-2"(FALSE) -> ()
                        n456 = Unbundle(w481) -> ("DESCRIPTION"=w473:string)  [unwired: 4 out]
                        n457 = Unbundle(w487) -> ("CYCLE"=w486:dbl, "MINS"=w485:dbl, "STATUS"=w470:string)
                        n458 = Get Date/Time String(seconds (now)=w483) -> (date string=w475:string, time string=w474:string)  [unwired: 2 in]
                        n459 = local read "LOG LAB04-2"() -> (w479:string)
                        n460 = Number To Fractional String(number=w485, precision (6)=2) -> (F-format string=w471:string)  [unwired: 2 in]
                        n461 = Number To Decimal String(number=w486) -> (decimal integer string=w472:string)  [unwired: 1 in]
                        n462 = Bundle(w476, "date string"=w475, "time string"=w474, "DESCRIPTION"=w473, w472, w471, "STATUS"=w470) -> (w469:T7)  [unwired: 1 in]
                        n463 = Concatenate Strings(w476, w480, w475, w480, w474, w480, w473, w480, w472, w480, w471, w480, w470, "\r\n") -> (w477:string)
                        n464 = Concatenate Strings(w479, w477) -> (w478:string)
                        n465 = local write "LOG LAB04-2"(w478) -> ()
                        n466 = call "sub vi - Log udate V1.vi"("data"=w469, "panel id"=w476) -> ("error out"=w468:errorcluster)  [unwired: 9 in]
                        n467 = local write "error out"(w468) -> ()
                      }
                    }
                  }
                }
                n468 = case shown="True" w454 {
                  frame False {
                  }
                  frame True {
                    n469 = local write "LF4-2"(TRUE) -> ()
                  }
                }
              }
              frame #8 {
                n470 = local read "RUN LAB05-1"() -> (w491:bool)
                n471 = local read "LF5-1"() -> (w493:bool)
                n472 = Not(x=w491) -> (.not. x?=w494:bool)
                n473 = And(x=w494, y=w493) -> (x .and. y?=w492:bool)
                n474 = case shown="True" w492 {
                  tunnel: w490 -> [_ w495]
                  frame False {
                  }
                  frame True {
                    n475 = stacked-sequence {
                      tunnel: w495 -> [w496 _]
                      frame #0 {
                        n476 = flat-sequence {
                          tunnel: [w498] -> w497
                          tunnel: w497 -> [w501]
                          tunnel: w496 -> [w500]
                          frame #0 {
                            n477 = local read "log5-1"() -> (w499:dbl)
                            n478 = Increment(x=w499) -> (x+1=w498:dbl)
                            n479 = local write "log5-1"(w498) -> ()
                          }
                          frame #1 {
                            n480 = Greater?(x=w501, y=w500) -> (0:w502:bool)
                            n481 = case shown="True" w502 {
                              frame False {
                              }
                              frame True {
                                n482 = local write "LOG LAB05-1"("") -> ()
                                n483 = local write "log5-1"(0) -> ()
                              }
                            }
                          }
                        }
                      }
                      frame #1 {
                        w513 = "LAB05-1"
                        w517 = "/"
                        n484 = local read "DISP LAB05-1"() -> (w524:T4)
                        n485 = local read "SET LAB05-1"() -> (w518:T5)
                        n486 = Get Date/Time In Seconds() -> (seconds since 1Jan1904=w520:timestamp)
                        n487 = local write "LF5-1"(FALSE) -> ()
                        n488 = Unbundle(w518) -> ("DESCRIPTION"=w510:string)  [unwired: 4 out]
                        n489 = Unbundle(w524) -> ("CYCLE"=w523:dbl, "MINS"=w522:dbl, "STATUS"=w507:string)
                        n490 = Get Date/Time String(seconds (now)=w520) -> (date string=w512:string, time string=w511:string)  [unwired: 2 in]
                        n491 = local read "LOG LAB05-1"() -> (w516:string)
                        n492 = Number To Fractional String(number=w522, precision (6)=2) -> (F-format string=w508:string)  [unwired: 2 in]
                        n493 = Number To Decimal String(number=w523) -> (decimal integer string=w509:string)  [unwired: 1 in]
                        n494 = Bundle(w513, "date string"=w512, "time string"=w511, "DESCRIPTION"=w510, w509, w508, "STATUS"=w507) -> (w506:T7)  [unwired: 1 in]
                        n495 = Concatenate Strings(w513, w517, w512, w517, w511, w517, w510, w517, w509, w517, w508, w517, w507, "\r\n") -> (w514:string)
                        n496 = Concatenate Strings(w516, w514) -> (w515:string)
                        n497 = local write "LOG LAB05-1"(w515) -> ()
                        n498 = call "sub vi - Log udate V1.vi"("data"=w506, "panel id"=w513) -> ("error out"=w505:errorcluster)  [unwired: 9 in]
                        n499 = local write "error out"(w505) -> ()
                      }
                    }
                  }
                }
                n500 = case shown="True" w491 {
                  frame False {
                  }
                  frame True {
                    n501 = local write "LF5-1"(TRUE) -> ()
                  }
                }
              }
              frame #9 {
                n502 = local read "RUN LAB05-2"() -> (w528:bool)
                n503 = local read "LF5-2"() -> (w530:bool)
                n504 = Not(x=w528) -> (.not. x?=w531:bool)
                n505 = And(x=w531, y=w530) -> (x .and. y?=w529:bool)
                n506 = case shown="True" w529 {
                  tunnel: w527 -> [_ w532]
                  frame False {
                  }
                  frame True {
                    n507 = stacked-sequence {
                      tunnel: w532 -> [w533 _]
                      frame #0 {
                        n508 = flat-sequence {
                          tunnel: [w535] -> w534
                          tunnel: w534 -> [w538]
                          tunnel: w533 -> [w537]
                          frame #0 {
                            n509 = local read "log5-2"() -> (w536:dbl)
                            n510 = Increment(x=w536) -> (x+1=w535:dbl)
                            n511 = local write "log5-2"(w535) -> ()
                          }
                          frame #1 {
                            n512 = Greater?(x=w538, y=w537) -> (0:w539:bool)
                            n513 = case shown="True" w539 {
                              frame False {
                              }
                              frame True {
                                n514 = local write "LOG LAB05-2"("") -> ()
                                n515 = local write "log5-2"(0) -> ()
                              }
                            }
                          }
                        }
                      }
                      frame #1 {
                        w550 = "LAB05-2"
                        w554 = "/"
                        n516 = local read "DISP LAB05-2"() -> (w561:T4)
                        n517 = local read "SET LAB05-2"() -> (w555:T5)
                        n518 = Get Date/Time In Seconds() -> (seconds since 1Jan1904=w557:timestamp)
                        n519 = local write "LF5-2"(FALSE) -> ()
                        n520 = Unbundle(w555) -> ("DESCRIPTION"=w547:string)  [unwired: 4 out]
                        n521 = Unbundle(w561) -> ("CYCLE"=w560:dbl, "MINS"=w559:dbl, "STATUS"=w544:string)
                        n522 = Get Date/Time String(seconds (now)=w557) -> (date string=w549:string, time string=w548:string)  [unwired: 2 in]
                        n523 = local read "LOG LAB05-2"() -> (w553:string)
                        n524 = Number To Fractional String(number=w559, precision (6)=2) -> (F-format string=w545:string)  [unwired: 2 in]
                        n525 = Number To Decimal String(number=w560) -> (decimal integer string=w546:string)  [unwired: 1 in]
                        n526 = Bundle(w550, "date string"=w549, "time string"=w548, "DESCRIPTION"=w547, w546, w545, "STATUS"=w544) -> (w543:T7)  [unwired: 1 in]
                        n527 = Concatenate Strings(w550, w554, w549, w554, w548, w554, w547, w554, w546, w554, w545, w554, w544, "\r\n") -> (w551:string)
                        n528 = Concatenate Strings(w553, w551) -> (w552:string)
                        n529 = local write "LOG LAB05-2"(w552) -> ()
                        n530 = call "sub vi - Log udate V1.vi"("data"=w543, "panel id"=w550) -> ("error out"=w542:errorcluster)  [unwired: 9 in]
                        n531 = local write "error out"(w542) -> ()
                      }
                    }
                  }
                }
                n532 = case shown="True" w528 {
                  frame False {
                  }
                  frame True {
                    n533 = local write "LF5-2"(TRUE) -> ()
                  }
                }
              }
            }
          }
          frame #3 {
            # "save current log files to network dir for viewing"
            # "save last months log files to networ dir for new month"
            # "send log data to main program"
            n534 = local read "LOG LAB05-2"() -> (w578:string)
            n535 = local read "LOG LAB02-1"() -> (w585:string)
            n536 = local read "LOG LAB03-2"() -> (w582:string)
            n537 = local read "LOG LAB04-1"() -> (w581:string)
            n538 = local read "LOG LAB05-1"() -> (w579:string)
            n539 = local read "LOG LAB02-2"() -> (w584:string)
            n540 = local read "LOG LAB04-2"() -> (w580:string)
            n541 = local read "LOG LAB03-1"() -> (w583:string)
            n542 = local read "LOG LAB01-2"() -> (w586:string)
            n543 = local read "LOG LAB01-1"() -> (w587:string)
            n544 = global write "Global display 3.vi" "log 5-2"(w578) -> ()
            n545 = global write "Global display 3.vi" "log 4-2"(w580) -> ()
            n546 = global write "Global display 3.vi" "log 1-1"(w587) -> ()
            n547 = global write "Global display 3.vi" "log 5-1"(w579) -> ()
            n548 = global write "Global display 3.vi" "log 1-2"(w586) -> ()
            n549 = global write "Global display 3.vi" "log 4-1"(w581) -> ()
            n550 = global write "Global display 3.vi" "log 2-2"(w584) -> ()
            n551 = global write "Global display 3.vi" "log 2-1"(w585) -> ()
            n552 = global write "Global display 3.vi" "log 3-1"(w583) -> ()
            n553 = global write "Global display 3.vi" "log 3-2"(w582) -> ()
            n554 = property on="Tab Control 2" class="TabCtl (strict)"() -> ("Pages"=w567:refnum<vi>[])  [unwired: 2 in, 2 out]
            n555 = global read "Global display 3.vi" "admin"() -> (w564:bool)
            n556 = Index Array(array=w567, index=8) -> (element=w565:refnum<vi>)
            n557 = property class="Page"(reference=w565, "PageVis"=w564) -> ()  [unwired: 1 in, 2 out]
            n558 = Get Date/Time In Seconds() -> (seconds since 1Jan1904=w575:timestamp)
            n559 = case shown="True" "Save Log Files\nTo Disk For\nViewing" {
              frame False {
              }
              frame True {
                n560 = stacked-sequence {
                  seq-local: [w592 _] -> [_ w595]
                  frame #0 {
                    n561 = call "sub vi - save log files V1.vi"() -> ("network dir"=w592:string)  [unwired: 10 in]
                  }
                  frame #1 {
                    n562 = local write "Save Log Files\nTo Disk For\nViewing"(FALSE) -> ()
                    n563 = Concatenate Strings("Saved:", w595) -> (w594:string)
                    n564 = One Button Dialog(message=w594) -> ()  [unwired: 1 in, 1 out]
                  }
                }
              }
            }
            n565 = Format Date/Time String(time format string (%c)="\\LabPanel%Y\\%b", seconds (now)=w575) -> (date/time string=w568:string)  [unwired: 1 in]
            n566 = local read "log file dir"() -> (w572:string)
            n567 = Equal?(x=w572, y="") -> (x = y?=w573:bool)
            n568 = Select(t=w568, s=w573, f=w572) -> (s? t:f=→"log file dir":string)
            n569 = local read "log file dir"() -> (w569:string)
            n570 = Not Equal?(x=w568, y=w569) -> (x != y?=w570:bool)
            n571 = case shown="True" w570 {
              tunnel: w569 -> [_ w589]
              tunnel: w568 -> [_ w588]
              frame False {
              }
              frame True {
                n572 = stacked-sequence {
                  tunnel: w589 -> [w590 _]
                  tunnel: w588 -> [_ w591]
                  frame #0 {
                    n573 = call "sub vi - save log dir V1.vi"("Dir Input"=w590) -> ()  [unwired: 11 in]
                  }
                  frame #1 {
                    n574 = local write "log file dir"(w591) -> ()
                  }
                }
              }
            }
          }
        }
        n575 = global read "Global display 1.vi" "stop disp"() -> (w2:bool)
        n576 = Or(x="Stop Button", y=w2) -> (x .or. y?=w4:bool)
      }
    }
  }
